vi "replaceAmountToken.vi"(8 "error in (no error)":errorcluster, 10 "Query In":string, 11 "Category in":refnum<class "Category.lvclass">) -> (0 "error out":errorcluster, 2 "Query Out":string, 3 "Category out":refnum<class "Category.lvclass">)   [LabVIEW 2018, in "Category.lvclass"]
uses:
  Category.lvclass
  Category.lvclass/Category.ctl
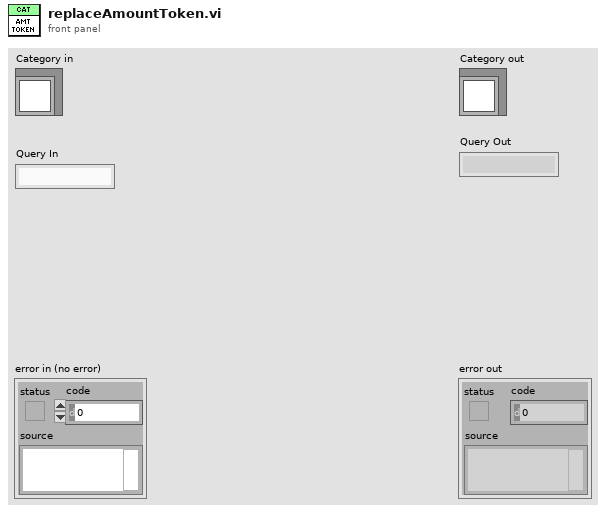
[diagram p1: front panel]
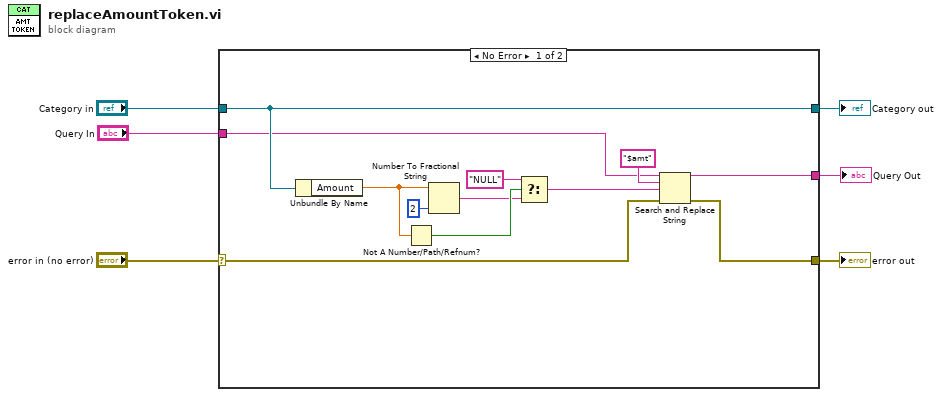
[diagram p0: block diagram]
diagram:
  n1 = case shown="No Error" "error in (no error)" {
    selector: "error in (no error)" -> [w8 w20]
    tunnel: [w7 w20] -> w5
    tunnel: [w13 w19] -> w3
    tunnel: "Category in" -> [w13 w19]
    tunnel: "Query In" -> [w10 _]
    tunnel: [w9 _] -> w1
    frame No Error {
      n2 = Unbundle By Name(w13) -> ("Amount"=w12:dbl)
      n3 = Not A Number/Path/Refnum?(number/path/refnum=w12) -> (NaN/Path/Refnum?=w16:bool)
      n4 = Number To Fractional String(number=w12, precision (6)=i16 2) -> (F-format string=w15:string)  [unwired: 2 in]
      n5 = Select(t="NULL", s=w16, f=w15) -> (s? t:f=w11:string)
      n6 = Search and Replace String(input string=w10, search string="$amt", replace string=w11, error in=w8) -> (result string=w9:string, error out=w7:errorcluster)  [unwired: 4 in, 2 out]
    }
    frame Error {
    }
  }
  "error out" <- w5
  "Category out" <- w3
  "Query Out" <- w1
